vi "송신신호.vi"() -> ()   [LabVIEW 2017]
panel:
  out "TX.CH1 2":waveform(dbl)(graph)
  out "Hz/1STEP":dbl
  in  "Bandwidth":dbl=40000.0 format="%#_6p"
  in  "초기 위상":dbl format="%#_13g"
  in  "STEP":i32=100
  out "TX Spectrum":cluster{"f0":dbl, "df":dbl, "magnitude":dbl[]}(graph)
  out "TX.CH1":waveform(dbl)(graph)
  in  "sampling rate":dbl=3760000.0 caption="Sampling Frequency" format="%0.2f"
  in  "Pulse length(sec)":dbl=4e-06 format="%#_6p"
  in  "Start Frequency(Hz)":dbl=430000.0 format="%#_6p"
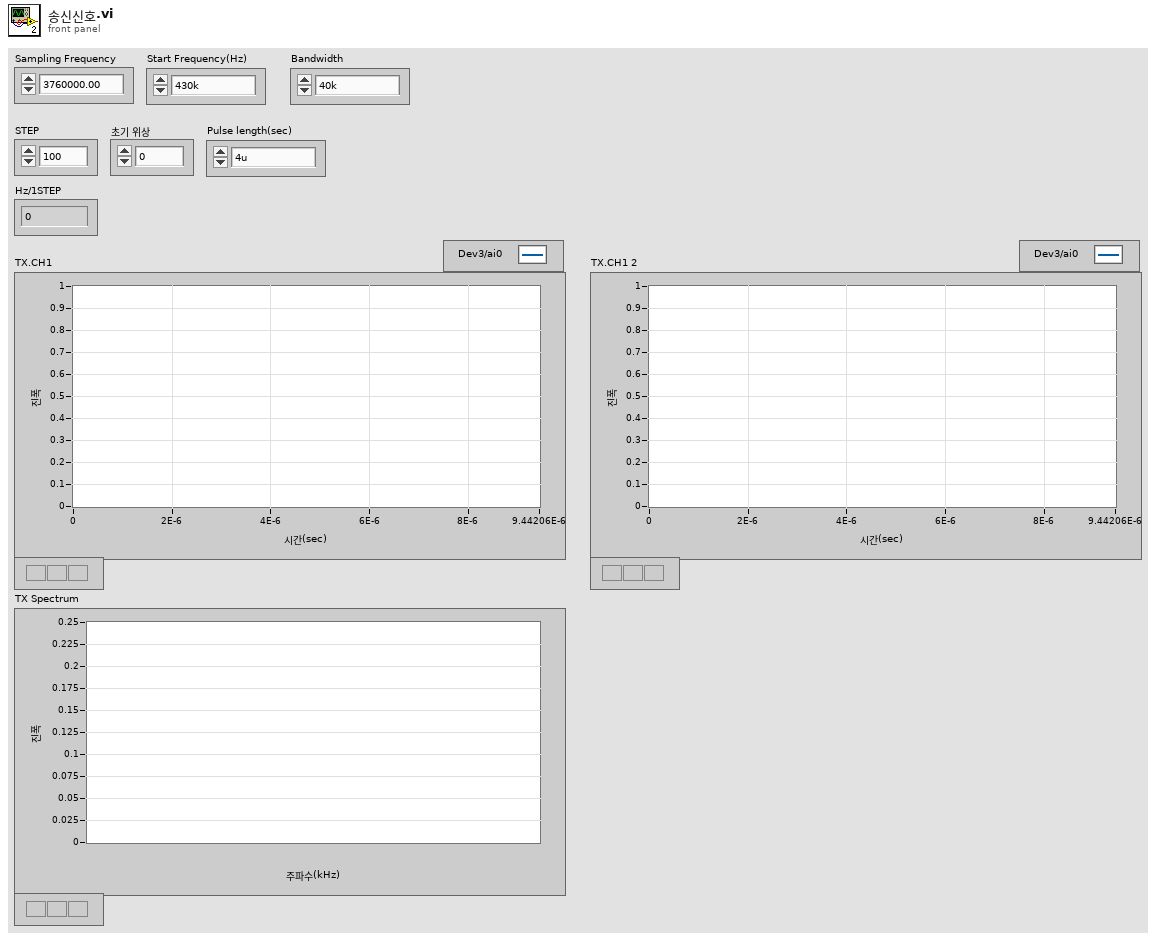
[diagram p1: front panel]
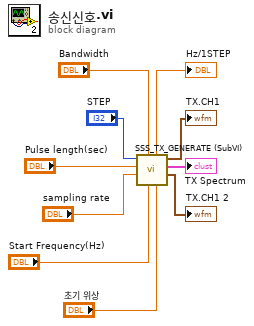
[diagram p0: block diagram]
diagram:
  n1 = call "SSS_TX_GENERATE (SubVI).vi"("초기 위상"="초기 위상", "Start Frequency(Hz)"="Start Frequency(Hz)", "Bandwidth"="Bandwidth", "sampling rate"="sampling rate", "Pulse length(sec)"="Pulse length(sec)", "STEP"="STEP") -> ("TX.CH1 2"=→"TX.CH1 2":waveform(dbl), "TX Spectrum"=→"TX Spectrum":cluster{"f0":dbl, "df":dbl, "magnitude":dbl[]}, "TX.CH1"=→"TX.CH1":waveform(dbl), "Hz/1STEP"=→"Hz/1STEP":dbl)  [unwired: 2 in]
